vi "AxisGoHome.vi"(8 "error in (no error)":errorcluster, 11 "ZanClass in":refnum<class "ZanClass.lvclass">) -> (0 "error out":errorcluster, 3 "ZanClass out":refnum<class "ZanClass.lvclass">)   [LabVIEW 2019, in "ZanClass.lvclass"]
uses:
  ZanClass.lvclass
  LLB/zmotion/zaux/zauxdll.lvlib
panel:
  in  "imode":i32
  in  "Creep":sgl
  in  "Speed":sgl
  in  "iaxis":i32
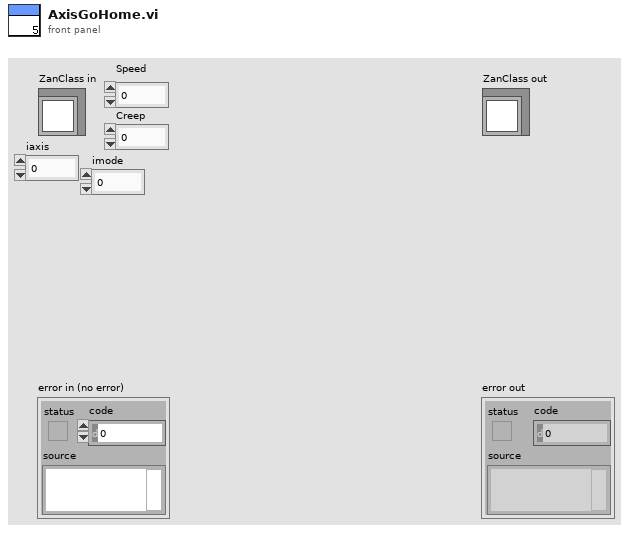
[diagram p1: front panel]
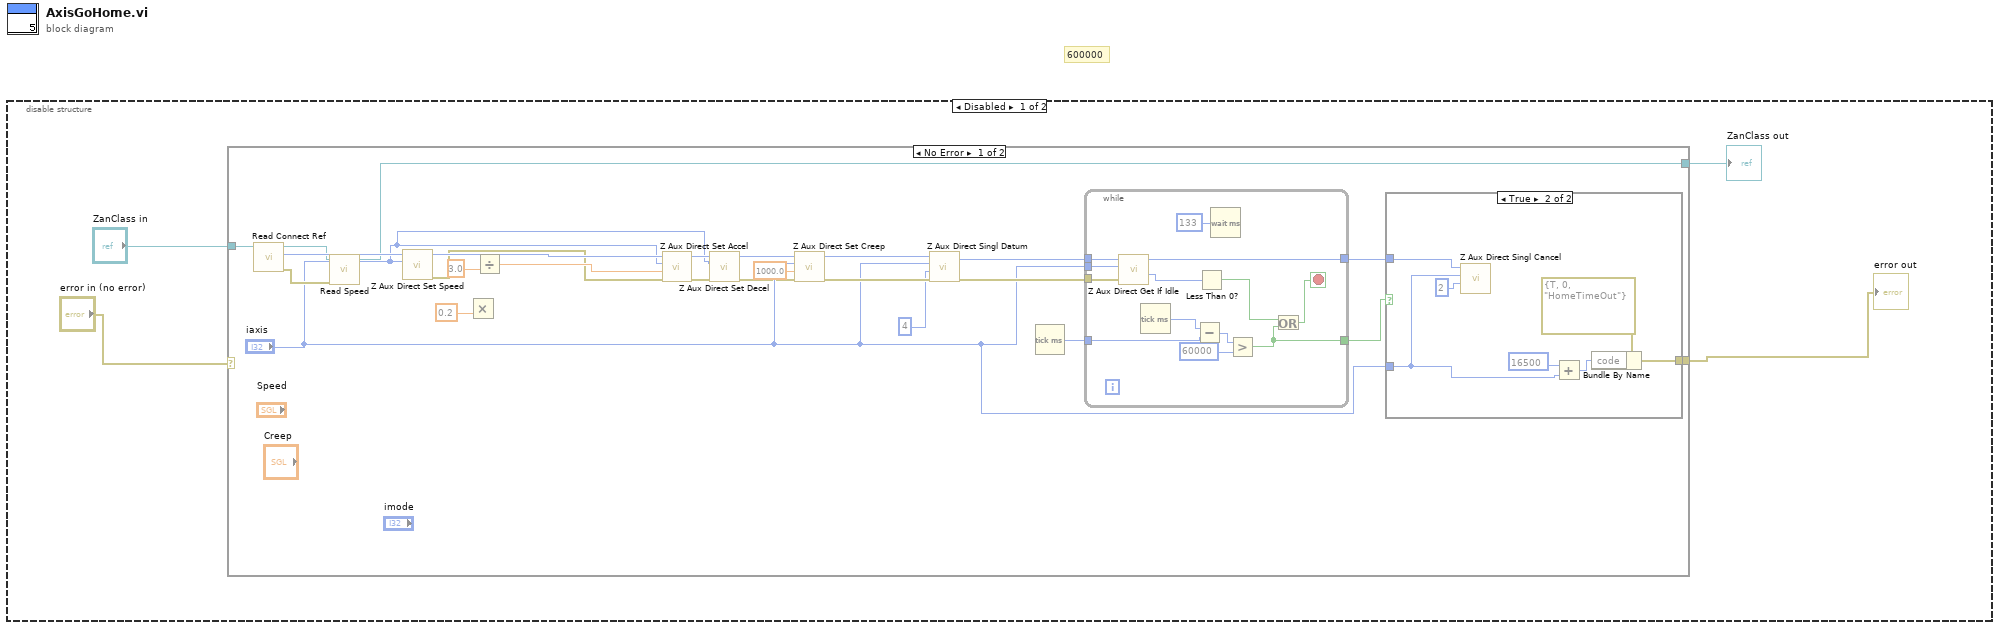
[diagram p0: block diagram]
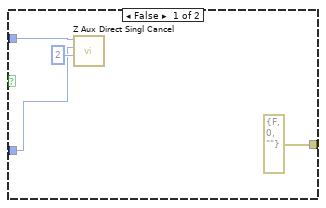
[diagram p2: hidden frame]
diagram:
  # "600000"
  n1 = disable-structure shown="Disabled" {
    frame Disabled {
      n2 = case shown="No Error" "error in (no error)" {
        selector: "error in (no error)" -> [_ w54]
        tunnel: "ZanClass in" -> [w29 w55]
        tunnel: [w19 w55] -> w2
        tunnel: [w20 w54] -> w1
        frame No Error {
          n3 = call-dynamic "Read Connect Ref.vi"("ZanClass in"=w29) -> ("error out"=w17:errorcluster, "CardHandle"=w28:i32, "ZanClass out"=w18:refnum<class "ZanClass.lvclass">)  [unwired: 7 in, 1 out]
          n4 = call-dynamic "Read Speed.vi"("error in (no error)"=w17, "AxisCard in"=w18) -> ("AxisCard out"=w19:refnum<class "ZanClass.lvclass">)  [unwired: 7 in, 2 out]
          n5 = call "Z Aux Direct Set Speed.vi"("iaxis"="iaxis", "handle"=w28) -> ("error out"=w8:errorcluster, "handle out"=w13:u32)  [unwired: 7 in, 1 out]
          n6 = Multiply(y=0.2) -> ()  [unwired: 1 in, 1 out]
          n7 = Divide(y=3.0) -> (x/y=w9:dbl)  [unwired: 1 in]
          n8 = call "Z Aux Direct Set Accel.vi"("error in (no error)"=w8, "fValue"=w9, "iaxis"="iaxis", "handle"=w13) -> ("error out"=w7:errorcluster, "handle out"=w14:u32)  [unwired: 5 in, 1 out]
          n9 = call "Z Aux Direct Set Decel.vi"("error in (no error)"=w7, "iaxis"="iaxis", "handle"=w14) -> ("error out"=w6:errorcluster, "handle out"=w12:u32)  [unwired: 6 in, 1 out]
          n10 = call "Z Aux Direct Set Creep.vi"("error in (no error)"=w6, "fValue"=sgl 1000.0, "iaxis"="iaxis", "handle"=w12) -> ("error out"=w26:errorcluster, "handle out"=w27:u32)  [unwired: 5 in, 1 out]
          n11 = call "Z Aux Direct Singl Datum.vi"("error in (no error)"=w26, "imode"=4, "iaxis"="iaxis", "handle"=w27) -> ("error out"=w21:errorcluster, "handle out"=w25:u32)  [unwired: 5 in, 1 out]
          n12 = Tick Count (ms)() -> (millisecond timer value=w24:u32)
          n13 = while {
            tunnel: w25 -> [w53]
            tunnel: "iaxis" -> [w52]
            tunnel: w24 -> [w48]
            tunnel: [w43] -> w23
            tunnel: [w42] -> w22
            tunnel: w21 -> [w41]
            stop <- w44 stop-if-true
            n14 = call "Z Aux Direct Get If Idle.vi"("error in (no error)"=w41, "iaxis"=w52, "handle"=w53) -> ("piValue out"=w51:i32, "handle out"=w42:u32)  [unwired: 5 in, 2 out]
            n15 = Tick Count (ms)() -> (millisecond timer value=w49:u32)
            n16 = Subtract(x=w49, y=w48) -> (x-y=w47:u32)
            n17 = Less Than 0?(x=w51) -> (x < 0?=w45:bool)
            n18 = Wait (ms)(milliseconds to wait=u32 133) -> ()  [unwired: 1 out]
            n19 = Greater?(x=w47, y=u32 60000) -> (0:w43:bool)
            n20 = Or(x=w45, y=w43) -> (x .or. y?=w44:bool)
          }
          n21 = case shown="True" w23 {
            tunnel: w22 -> [w32 w40]
            tunnel: "iaxis" -> [w31 w34]
            tunnel: [errorcluster {"status"=FALSE, "code"=0, "source"=""} ("error constant") w37] -> w20
            frame False {
              n22 = call "Z Aux Direct Singl Cancel.vi"("imode"=2, "iaxis"=w31, "handle"=w32) -> ()  [unwired: 6 in, 3 out]
            }
            frame True {
              n23 = call "Z Aux Direct Singl Cancel.vi"("imode"=2, "iaxis"=w34, "handle"=w40) -> ()  [unwired: 6 in, 3 out]
              n24 = Add(x=16500, y=w34) -> (x+y=w35:i32)
              n25 = Bundle By Name(cluster=errorcluster {"status"=TRUE, "code"=0, "source"="HomeTimeOut"} ("error constant"), "code"=w35) -> (w37:errorcluster)
            }
          }
        }
        frame Error {
        }
      }
      "error out" <- w1
      "ZanClass out" <- w2
    }
    frame Enabled {
    }
  }
